vi "HFRR ADV v01.vi"() -> ()   [LabVIEW 2025] (continued)
            n1565 = Concatenate Strings("(" ("string"), w1652, " ) % RH," ("string")) -> (w1651:string)
            n1566 = Concatenate Strings("(" ("string"), w1648, ")  Deg C ," ("string")) -> (w1647:string)
            n1567 = Concatenate Strings("(" ("string"), w1645, ")  Microns," ("string")) -> (w1644:string)
            n1568 = Concatenate Strings("(" ("string"), w1641, ")  kPa," ("string")) -> (w1631:string)
            n1569 = Concatenate Strings(w1685, ".dwm" ("Substring")) -> (w1683:string)
            n1570 = String To Path(string=w1683) -> (path=w1682:path)
            n1571 = Concatenate Strings(w1665, w1630, " Humidity before test= " ("Substring"), w1660, w1630, " Temperature before test = " ("Substring"), w1655, w1630, " Humidity after test= " ("Substring"), w1651, w1630, "Temperature after test = " ("Substring"), w1647, w1630, "MSD = " ("Substring"), w1644, w1630, "  AVP = " ("Substring"), w1631, w1630, "  HCF                     =( " ("Substring"), w1637, w1630, " WS1.4                  = " ("Substring"), w1633, w1630) -> (w1629:string)
            "data" <- w1629
            n1572 = call <vilib>:"Write Characters To File.vi"("append to file? (new file:F)"=FALSE, "character string"=w1629, "file path (dialog if empty)"=w1682) -> ()  [unwired: 2 in, 1 out]
            n1573 = Match Pattern(string=w1629, regular expression="!") -> (after substring=→"export":string)  [unwired: 1 in, 3 out]
          }
        }
        n1574 = Add(x=231.864, y=w1601) -> (x+y=w1598:dbl)
        n1575 = Add(x=231.864, y=w1614) -> (x+y=w1611:dbl)
        n1576 = Divide(x=1705.984, y=w1598) -> (x/y=w1599:dbl)
        n1577 = Divide(x=1705.984, y=w1611) -> (x/y=w1612:dbl)
        n1578 = local read "Humidity before test"() -> (w1603:dbl)
        n1579 = local read "Humidity after test"() -> (w1616:dbl)
        n1580 = Subtract(x=8.017352 ("y"), y=w1599) -> (x-y=w1625:dbl)
        n1581 = Subtract(x=8.017352 ("y"), y=w1612) -> (x-y=w1619:dbl)
        n1582 = expression code="10**y"(w1625) -> (w1605:dbl)
        n1583 = expression code="10**y"(w1619) -> (w1618:dbl)
        n1584 = Multiply(x=w1603, y=w1605) -> (x*y=w1604:dbl)
        n1585 = Multiply(x=w1616, y=w1618) -> (x*y=w1617:dbl)
        n1586 = Divide(x=w1604, y=750.0) -> (x/y=w1620:dbl)
        n1587 = Divide(x=w1617, y=750.0) -> (x/y=w1621:dbl)
        n1588 = Add(x=w1620, y=w1621) -> (x+y=w1622:dbl)
        n1589 = Divide(x=w1622, y=2.0) -> (x/y=w1624:dbl)
        n1590 = local write "AVP"(w1624) -> ()
        n1591 = Subtract(x=1.4, y=w1624) -> (x-y=w1607:dbl)
        n1592 = local read "HCF"() -> (w1608:dbl)
      }
      frame Enabled {
      }
    }
    n1593 = case shown="True" "EDIT 3" {
      frame False {
      }
      frame True {
        n1594 = local write "EDIT 3"(FALSE ("EDIT 3")) -> ()
        n1595 = local write "Main Tab"(T2."About" ("Main Tab")) -> ()
      }
    }
    n1596 = case shown="True" w1579 {
      frame False {
      }
      frame True {
        n1597 = local write "Re-Initialise"(FALSE ("Re-Initialise")) -> ()
      }
    }
    n1598 = case shown="False" w1593 {
      frame False {
        n1599 = local read "stopT"() -> (w2573:bool)
        n1600 = case shown="True" w2573 {
          frame False {
          }
          frame True {
            n1601 = local write "stopT"(FALSE) -> ()
          }
        }
      }
      frame True {
        "stopT" <- TRUE
      }
    }
    n1602 = case shown="False" w1591 {
      frame False {
      }
      frame True {
      }
    }
    n1603 = case shown="True" w1581 {
      frame False {
        n1604 = property on="Password 2" class="Str"("Visible"=FALSE) -> ()  [unwired: 2 in, 2 out]
        n1605 = local write "Password 2"("" ("Password")) -> ()
      }
      frame True {
        n1606 = property on="Password 2" class="Str"("Visible"=TRUE) -> ()  [unwired: 2 in, 2 out]
        n1607 = Equal?(x="Password 2", y="HFRR1234") -> (x = y?=w1714:bool)
        n1608 = case shown="True" w1714 {
          tunnel: "Password 2" -> [w1717 _]
          frame False {
            n1609 = String Length(string=w1717) -> (length=w1718:i32)
            n1610 = Greater Than 0?(x=w1718) -> (x > 0?=w1716:bool)
            n1611 = case shown="False" w1716 {
              frame False {
                n1612 = property on="Password 2" class="Str"("Caption.Text"="Password (Advance Setting)") -> ()  [unwired: 2 in, 2 out]
              }
              frame True {
                n1613 = property on="Password 2" class="Str"("Caption.Text"="Incorrect Password!") -> ()  [unwired: 2 in, 2 out]
              }
            }
          }
          frame True {
            n1614 = local write "EDIT 2"(FALSE ("EDIT 2")) -> ()
            n1615 = local write "Password 2"("" ("Password")) -> ()
            n1616 = local write "Main Tab"(T2."Advance" ("Main Tab")) -> ()
            n1617 = local write "Main Dashboard Buttons"(T1."Advance" ("Main Dashboard Buttons")) -> ()
          }
        }
      }
    }
    n1618 = case shown="True" "Prog Uno" {
      frame False {
      }
      frame True {
        n1619 = stacked-sequence {
          frame #0 {
            n1620 = Delete(path (use dialog)=path "C:/LAB-IQ-NXT/UNOCOMPILE.bat" ("working directory")) -> ()  [unwired: 4 in, 3 out]
          }
          frame #1 {
            n1621 = local read "Com Port 1"() -> (w2179:refnum<visa-resource-name>)
            n1622 = Concatenate Strings("cmd.exe /c \"mode " ("command line"), w2179, ":1200,n,8,1\"\n" ("command line")) -> (w2184:string)
            n1623 = Concatenate Strings(w2184, "CD\\\nCD WinDucom\navrdude -C avrdude.conf -v -patmega328p -carduino -P" ("command line"), w2179, " -b115200 -D -Uflash:w:UNO_V20.hex:i\n" ("command line"), "\r") -> (w2186:string)
            "STR" <- w2186
            n1624 = call <vilib>:"Write Characters To File.vi"("append to file? (new file:F)"=FALSE, "character string"=w2186, "file path (dialog if empty)"=path "C:/LAB-IQ/UNOCOMPILE.bat" ("working directory")) -> ()  [unwired: 2 in, 1 out]
          }
          frame #2 {
            n1625 = disable-structure shown="Disabled" {
              frame Disabled {
                w2190 = "cmd.exe  /c \"C:\\LAB-IQ-NXT\\UNOCOMPILE.bat\"" ("string")
                n1626 = local write "Prog Uno"(FALSE ("run minimized? (F)")) -> ()
                n1627 = call <vilib>:"System Exec.vi"("expected output size  (4096)"=u32 65535, "run minimized? (F)"=FALSE, "wait until completion? (T)"=TRUE ("run minimized? (F)"), "working directory"=path "C:/LAB-IQ-NXT", "standard input"=w2190, "command line"=w2190) -> ("error out"=w2189:errorcluster, "standard output"=→"String 42":string)  [unwired: 2 in, 2 out]
                "error out 3" <- w2189
                n1628 = flat-sequence {
                  tunnel: w2189 -> [_]
                  frame #0 {
                  }
                }
              }
              frame Enabled {
              }
            }
          }
        }
      }
    }
    n1629 = case shown="\"CEC F-096-A-06\"" "TEST STANDARD" {
      tunnel: [2.0 ("Set Temp") 0.0 ("Set Temp") 2.0 ("Set Temp") 0.0 ("Set Temp")] -> w1582
      frame "ASTM D6079", Default {
        w2136 = 50.0 ("Hz")
        w2137 = 53.0 ("Set Rh")
        w2139 = 1.0 ("Set Strk")
        w2138 = 60.0 ("Set Temp")
        # "astm hide"
        n1630 = local write "NORMAL LOAD"(200.0 ("NORMAL LOAD")) -> ()
        n1631 = local write "Set Strk"(w2139) -> ()
        n1632 = local write "Set Hz"(w2136) -> ()
        n1633 = local write "Set Temp"(w2138) -> ()
        n1634 = local write "Set Rh"(w2137) -> ()
        n1635 = local write "test time"(75.0 ("test time")) -> ()
        n1636 = local write "Set Stroke:"(w2139) -> ()
        n1637 = local write "Set Humidity:"(w2137) -> ()
        n1638 = local write "Set Frequency:"(w2136) -> ()
        n1639 = local write "Set Temperature:"(w2138) -> ()
        "Test Standard" <- "ASTM D6079" ("Test Standard 2")
      }
      frame "ISO 12156" {
        n1640 = local write "Set Strk"(1.0 ("Set Strk")) -> ()
        n1641 = local write "NORMAL LOAD"(200.0 ("NORMAL LOAD")) -> ()
        n1642 = local write "Set Temp"(60.0 ("Set Temp")) -> ()
        n1643 = local write "test time"(75.0 ("test time")) -> ()
        n1644 = local write "Set Hz"(50.0 ("Hz")) -> ()
        n1645 = local write "Set Rh"(53.0 ("Set Rh")) -> ()
      }
      frame "CEC F-096-A-06" {
        n1646 = local write "Set Strk"(1.0 ("Set Strk")) -> ()
        n1647 = local write "NORMAL LOAD"(200.0 ("NORMAL LOAD")) -> ()
        n1648 = local write "Set Temp"(60.0 ("Set Temp")) -> ()
        n1649 = local write "test time"(75.0 ("test time")) -> ()
        n1650 = local write "Set Hz"(50.0 ("Hz")) -> ()
        n1651 = local write "Set Rh"(53.0 ("Set Rh")) -> ()
      }
      frame "Custom" {
      }
    }
    n1652 = case shown="True" "Prog Due" {
      frame False {
      }
      frame True {
        n1653 = stacked-sequence {
          frame #0 {
            n1654 = Delete(path (use dialog)=path "C:/LAB-IQ/DUECOMPILE.bat" ("working directory")) -> ()  [unwired: 4 in, 3 out]
          }
          frame #1 {
            n1655 = disable-structure shown="Disabled" {
              frame Disabled {
                n1656 = local read "visa due"() -> (w2161:string)
                n1657 = Concatenate Strings("cmd.exe /c \"mode " ("command line"), w2161, ":1200,n,8,1\"\n" ("command line")) -> (w2166:string)
                n1658 = Concatenate Strings(w2166, "CD\\\nCD WinDucom\nTIMEOUT 1\n bossac.exe -i -d --port=" ("command line"), w2161, " -U false -e -w -v -b DUE.bin -R\n" ("command line"), "\r") -> (w2168:string)
                "concatenated string 2" <- w2168
                n1659 = call <vilib>:"Write Characters To File.vi"("append to file? (new file:F)"=FALSE, "character string"=w2168, "file path (dialog if empty)"=path "C:/LAB-IQ-NXT/DUECOMPILE.bat" ("working directory")) -> ()  [unwired: 2 in, 1 out]
              }
              frame Enabled {
              }
            }
          }
          frame #2 {
            # "C:\\LAB-IQ-NXT\\DUECOMPILE.bat"
            n1660 = disable-structure shown="Disabled" {
              frame Disabled {
                w2173 = "cmd.exe  /c \"C:\\LAB-IQ-NXT\\DUECOMPILE.bat\"" ("string")
                n1661 = call <vilib>:"System Exec.vi"("expected output size  (4096)"=u32 65535, "run minimized? (F)"=FALSE, "wait until completion? (T)"=TRUE ("run minimized? (F)"), "working directory"=path "C:/LAB-IQ-NXT", "standard input"=w2173, "command line"=w2173) -> ("error out"=w2172:errorcluster, "standard output"=→"String 44":string)  [unwired: 2 in, 2 out]
                "error out 4" <- w2172
                n1662 = flat-sequence {
                  tunnel: w2172 -> [_]
                  frame #0 {
                  }
                }
              }
              frame Enabled {
              }
            }
            n1663 = local write "Prog Due"(FALSE ("Prog Due")) -> ()
          }
        }
      }
    }
    n1664 = Or(x=w1578, y=w1576) -> (x .or. y?=w1577:bool)
    n1665 = case shown="\"About\"" w1575 {
      tunnel: [T22."Acquire" ("Main Tab") T22."Compare Files" ("Main Tab") T22."About" ("Main Tab")] -> w1589
      frame "Acquire", Default {
      }
      frame "Compare Files" {
      }
      frame "About" {
      }
    }
    n1666 = Or(x=w1583, y="OPEN") -> (x .or. y?=w1584:bool)
    n1667 = case shown="True" w1584 {
      tunnel: w1583 -> [_ w1725]
      frame False {
      }
      frame True {
        n1668 = stacked-sequence {
          tunnel: w1725 -> [_ w1792 _ _]
          frame #0 {
            w1741 = "  " ("String 6")
            n1669 = local write "OPEN"(FALSE ("open")) -> ()
            n1670 = local read "string1 2"() -> (w1729:string)
            n1671 = local read "string1 3"() -> (w1728:string)
            n1672 = local read "string1 4"() -> (w1727:string)
            n1673 = property on="OPEN" class="Bool (strict)"("Visible"=FALSE) -> ()  [unwired: 2 in, 2 out]
            n1674 = local write "String 6"(w1741) -> ()
            n1675 = local write "String 7"(w1741) -> ()
            n1676 = local write "String 8"(w1741) -> ()
            n1677 = local write "String 12"(w1741) -> ()
            n1678 = local read "OK Button 16"() -> (w1726:bool)
            n1679 = String To Path(string=w1729) -> (path=w1737:path)
            n1680 = String To Path(string=w1728) -> (path=w1736:path)
            n1681 = String To Path(string=w1727) -> (path=w1735:path)
            n1682 = case shown="True" w1726 {
              tunnel: [w1742 w1743] -> w1730
              frame False {
                n1683 = local read "string1"() -> (w1742:string)
              }
              frame True {
                n1684 = local read "String Indicator 4"() -> (w1743:string)
              }
            }
            n1685 = Open/Create/Replace File "Open File"(file path (use dialog)=w1737) -> (refnum out=w1733:refnum<file>)  [unwired: 5 in, 2 out]
            n1686 = Open/Create/Replace File "Open File"(file path (use dialog)=w1736) -> (refnum out=w1732:refnum<file>)  [unwired: 5 in, 2 out]
            n1687 = Open/Create/Replace File "Open File"(file path (use dialog)=w1735) -> (refnum out=w1731:refnum<file>)  [unwired: 5 in, 2 out]
            n1688 = while {
              tunnel: w1733 -> [w1755]
              i -> [w1751]
              stop <- w1750 continue-if-true
              (unwired) TRUE ("line mode (F)")
              n1689 = Read from Text File "Read File"(file (use dialog)=w1755) -> (text=w1752:string)  [unwired: 3 in, 3 out]
              n1690 = local write "Numeric 11"(w1751) -> ()
              n1691 = String Length(string=w1752) -> (length=w1754:i32)
              n1692 = Greater?(x=w1754, y=1) -> (0:w1750:bool)
            }
            n1693 = while {
              tunnel: w1732 -> [w1761]
              i -> [w1757]
              stop <- w1756 continue-if-true
              (unwired) TRUE ("line mode (F)")
              n1694 = Read from Text File "Read File"(file (use dialog)=w1761) -> (text=w1758:string)  [unwired: 3 in, 3 out]
              n1695 = local write "Numeric 12"(w1757) -> ()
              n1696 = String Length(string=w1758) -> (length=w1760:i32)
              n1697 = Greater?(x=w1760, y=1) -> (0:w1756:bool)
            }
            n1698 = while {
              tunnel: w1731 -> [w1767]
              i -> [w1763]
              stop <- w1762 continue-if-true
              (unwired) TRUE ("line mode (F)")
              n1699 = Read from Text File "Read File"(file (use dialog)=w1767) -> (text=w1764:string)  [unwired: 3 in, 3 out]
              n1700 = local write "Numeric 13"(w1763) -> ()
              n1701 = String Length(string=w1764) -> (length=w1766:i32)
              n1702 = Greater?(x=w1766, y=1) -> (0:w1762:bool)
            }
            n1703 = String To Path(string=w1730) -> (path=w1738:path)
            n1704 = Open/Create/Replace File "Open File"(file path (use dialog)=w1738) -> (refnum out=w1734:refnum<file>)  [unwired: 5 in, 2 out]
            n1705 = while {
              tunnel: w1734 -> [w1749]
              i -> [w1745]
              stop <- w1744 continue-if-true
              (unwired) TRUE ("line mode (F)")
              n1706 = Read from Text File "Read File"(file (use dialog)=w1749) -> (text=w1746:string)  [unwired: 3 in, 3 out]
              n1707 = local write "Numeric 8"(w1745) -> ()
              n1708 = String Length(string=w1746) -> (length=w1748:i32)
              n1709 = Greater?(x=w1748, y=1) -> (0:w1744:bool)
            }
          }
          frame #1 {
            w1919 = FALSE ("ACTUAL   MERGE")
            # "Sample Temp"
            # "ECR"
            # "COF"
            # "Time\nCOF\nFF\nTemp"
            n1710 = case shown="True" w1792 {
              tunnel: [w1939 w1940] -> w1793
              frame False {
                n1711 = local read "string1"() -> (w1939:string)
              }
              frame True {
                n1712 = local read "String Indicator 4"() -> (w1940:string)
              }
            }
            n1713 = local read "string1 3"() -> (w1837:string)
            n1714 = String To Path(string=w1793) -> (path=w1924:path)
            n1715 = String To Path(string=w1837) -> (path=w1935:path)
            n1716 = local read "Numeric 12"() -> (w1921:i32)
            n1717 = local read "Numeric 8"() -> (w1923:i32)
            n1718 = local read "string1 2"() -> (w1838:string)
            n1719 = local read "string1 4"() -> (w1836:string)
            n1720 = Open/Create/Replace File "Open File"(file path (use dialog)=w1924) -> (refnum out=w1938:refnum<file>, error out=w1937:errorcluster)  [unwired: 5 in, 1 out]
            n1721 = Open/Create/Replace File "Open File"(file path (use dialog)=w1935) -> (refnum out=w1931:refnum<file>, error out=w1932:errorcluster)  [unwired: 5 in, 1 out]
            n1722 = for {
              N: w1923 -> [_]
              tunnel: w1938 -> [w2086]
              tunnel: w1937 -> [w2085]
              tunnel: [w2075] -> w1850 mode=indexing
              tunnel: [w2073] -> w1907 mode=indexing
              tunnel: [w2074] -> w1902 mode=indexing
              tunnel: w1919 -> [_]
              tunnel: [w2067] -> w1904 mode=indexing
              tunnel: [w2063] -> w1873 mode=indexing
              tunnel: [w2059] -> w1848 mode=indexing
              tunnel: [w2055] -> w1829 mode=indexing
              tunnel: [w2050] -> w1789 mode=indexing
              (unwired) TRUE ("line mode (F)")
              # "freq"
              # "Stroke"
              # "Time"
              # "CoF"
              # "Humidity"
              # "Temp"
              # "Air Temp"
              # "ECR"
              n1723 = Read from Text File "Read File"(file (use dialog)=w2086, error in=w2085) -> (text=w2051:string)  [unwired: 2 in, 3 out]
              n1724 = local write "String 6"(w2051) -> ()
              n1725 = String Subset(string=w2051, offset (0)=0, length (rest)=14 ("length (rest)")) -> (substring=w2079:string)
              n1726 = String Subset(string=w2051, offset (0)=35, length (rest)=9 ("length (rest)")) -> (substring=w2076:string)
              n1727 = String Subset(string=w2051, offset (0)=15, length (rest)=9 ("length (rest)")) -> (substring=w2082:string)
              n1728 = Fract/Exp String To Number(string=w2079) -> (number=w2075:dbl)  [unwired: 3 in, 1 out]
              n1729 = Fract/Exp String To Number(string=w2076) -> (number=w2074:dbl)  [unwired: 3 in, 1 out]
              n1730 = Fract/Exp String To Number(string=w2082) -> (number=w2073:dbl)  [unwired: 3 in, 1 out]
              n1731 = String Subset(string=w2051, offset (0)=85, length (rest)=9 ("length (rest)")) -> (substring=w2052:string)
              n1732 = String Subset(string=w2051, offset (0)=25, length (rest)=9 ("length (rest)")) -> (substring=w2058:string)
              n1733 = String Subset(string=w2051, offset (0)=55, length (rest)=9 ("length (rest)")) -> (substring=w2060:string)
              n1734 = String Subset(string=w2051, offset (0)=45, length (rest)=9 ("length (rest)")) -> (substring=w2066:string)
              n1735 = String Subset(string=w2051, offset (0)=65, length (rest)=9 ("length (rest)")) -> (substring=w2072:string)
              n1736 = Fract/Exp String To Number(string=w2058) -> (number=w2055:dbl)  [unwired: 3 in, 1 out]
              n1737 = Fract/Exp String To Number(string=w2052) -> (number=w2050:dbl)  [unwired: 3 in, 1 out]
              n1738 = Fract/Exp String To Number(string=w2060) -> (number=w2059:dbl)  [unwired: 3 in, 1 out]
              n1739 = Fract/Exp String To Number(string=w2066) -> (number=w2063:dbl)  [unwired: 3 in, 1 out]
              n1740 = Fract/Exp String To Number(string=w2072) -> (number=w2069:dbl)  [unwired: 3 in, 1 out]
              n1741 = Add(x=w2069, y=0.0) -> (x+y=w2067:dbl)
            }
            n1742 = for {
              N: w1921 -> [_]
              tunnel: w1932 -> [w2012]
              tunnel: w1931 -> [w2011]
              tunnel: [w2001] -> w1890 mode=indexing
              tunnel: [w1999] -> w1888 mode=indexing
              tunnel: [w2000] -> w1884 mode=indexing
              tunnel: w1919 -> [_]
              tunnel: [w1993] -> w1886 mode=indexing
              tunnel: [w1989] -> w1868 mode=indexing
              tunnel: [w1985] -> w1844 mode=indexing
              tunnel: [w1982] -> w1825 mode=indexing
              tunnel: [w1978] -> w1784 mode=indexing
              (unwired) 9 ("length (rest)")
              (unwired) 9 ("length (rest)")
              (unwired) TRUE ("line mode (F)")
              n1743 = Read from Text File "Read File"(file (use dialog)=w2011, error in=w2012) -> (text=w1979:string)  [unwired: 2 in, 3 out]
              n1744 = local write "String 8"(w1979) -> ()
              n1745 = String Subset(string=w1979, offset (0)=85) -> (substring=w1981:string)  [unwired: 1 in]
              n1746 = String Subset(string=w1979, offset (0)=35, length (rest)=9 ("length (rest)")) -> (substring=w2002:string)
              n1747 = String Subset(string=w1979, offset (0)=55, length (rest)=9 ("length (rest)")) -> (substring=w1987:string)
              n1748 = String Subset(string=w1979, offset (0)=25) -> (substring=w1983:string)  [unwired: 1 in]
              n1749 = String Subset(string=w1979, offset (0)=15, length (rest)=9 ("length (rest)")) -> (substring=w2008:string)
              n1750 = String Subset(string=w1979, offset (0)=0, length (rest)=14 ("length (rest)")) -> (substring=w2005:string)
              n1751 = String Subset(string=w1979, offset (0)=45, length (rest)=9 ("length (rest)")) -> (substring=w1992:string)
              n1752 = String Subset(string=w1979, offset (0)=65, length (rest)=9 ("length (rest)")) -> (substring=w1998:string)
              n1753 = Fract/Exp String To Number(string=w1981) -> (number=w1978:dbl)  [unwired: 3 in, 1 out]
              n1754 = Fract/Exp String To Number(string=w2002) -> (number=w2000:dbl)  [unwired: 3 in, 1 out]
              n1755 = Fract/Exp String To Number(string=w1987) -> (number=w1985:dbl)  [unwired: 3 in, 1 out]
              n1756 = Fract/Exp String To Number(string=w1983) -> (number=w1982:dbl)  [unwired: 3 in, 1 out]
              n1757 = Fract/Exp String To Number(string=w2008) -> (number=w1999:dbl)  [unwired: 3 in, 1 out]
              n1758 = Fract/Exp String To Number(string=w2005) -> (number=w2001:dbl)  [unwired: 3 in, 1 out]
              n1759 = Fract/Exp String To Number(string=w1992) -> (number=w1989:dbl)  [unwired: 3 in, 1 out]
              n1760 = Fract/Exp String To Number(string=w1998) -> (number=w1995:dbl)  [unwired: 3 in, 1 out]
              n1761 = Add(x=w1995, y=0.0) -> (x+y=w1993:dbl)
            }
            n1762 = String To Path(string=w1838) -> (path=w1936:path)
            n1763 = String To Path(string=w1836) -> (path=w1930:path)
            n1764 = local read "Numeric 11"() -> (w1920:i32)
            n1765 = local read "Numeric 13"() -> (w1922:i32)
            n1766 = Open/Create/Replace File "Open File"(file path (use dialog)=w1936) -> (refnum out=w1934:refnum<file>, error out=w1933:errorcluster)  [unwired: 5 in, 1 out]
            n1767 = Open/Create/Replace File "Open File"(file path (use dialog)=w1930) -> (refnum out=w1929:refnum<file>, error out=w1928:errorcluster)  [unwired: 5 in, 1 out]
            n1768 = for {
              N: w1920 -> [_]
              tunnel: w1934 -> [w2049]
              tunnel: w1933 -> [w2048]
              tunnel: [w2038] -> w1900 mode=indexing
              tunnel: [w2036] -> w1898 mode=indexing
              tunnel: [w2037] -> w1893 mode=indexing
              tunnel: w1919 -> [_]
              tunnel: [w2030] -> w1895 mode=indexing
              tunnel: [w2026] -> w1871 mode=indexing
              tunnel: [w2022] -> w1846 mode=indexing
              tunnel: [w2018] -> w1827 mode=indexing
              tunnel: [w2013] -> w1785 mode=indexing
              (unwired) TRUE ("line mode (F)")
              n1769 = Read from Text File "Read File"(file (use dialog)=w2049, error in=w2048) -> (text=w2014:string)  [unwired: 2 in, 3 out]
              n1770 = local write "String 7"(w2014) -> ()
              n1771 = String Subset(string=w2014, offset (0)=85, length (rest)=9 ("length (rest)")) -> (substring=w2017:string)
              n1772 = String Subset(string=w2014, offset (0)=35, length (rest)=9 ("length (rest)")) -> (substring=w2039:string)
              n1773 = String Subset(string=w2014, offset (0)=55, length (rest)=9 ("length (rest)")) -> (substring=w2025:string)
              n1774 = String Subset(string=w2014, offset (0)=25, length (rest)=9 ("length (rest)")) -> (substring=w2019:string)
              n1775 = String Subset(string=w2014, offset (0)=45, length (rest)=9 ("length (rest)")) -> (substring=w2027:string)
              n1776 = String Subset(string=w2014, offset (0)=0, length (rest)=14 ("length (rest)")) -> (substring=w2042:string)
              n1777 = String Subset(string=w2014, offset (0)=15, length (rest)=9 ("length (rest)")) -> (substring=w2045:string)
              n1778 = String Subset(string=w2014, offset (0)=65, length (rest)=9 ("length (rest)")) -> (substring=w2031:string)
              n1779 = Fract/Exp String To Number(string=w2017) -> (number=w2013:dbl)  [unwired: 3 in, 1 out]
              n1780 = Fract/Exp String To Number(string=w2039) -> (number=w2037:dbl)  [unwired: 3 in, 1 out]
              n1781 = Fract/Exp String To Number(string=w2025) -> (number=w2022:dbl)  [unwired: 3 in, 1 out]
              n1782 = Fract/Exp String To Number(string=w2019) -> (number=w2018:dbl)  [unwired: 3 in, 1 out]
              n1783 = Fract/Exp String To Number(string=w2027) -> (number=w2026:dbl)  [unwired: 3 in, 1 out]
              n1784 = Fract/Exp String To Number(string=w2042) -> (number=w2038:dbl)  [unwired: 3 in, 1 out]
              n1785 = Fract/Exp String To Number(string=w2045) -> (number=w2036:dbl)  [unwired: 3 in, 1 out]
              n1786 = Fract/Exp String To Number(string=w2031) -> (number=w2034:dbl)  [unwired: 3 in, 1 out]
              n1787 = Add(x=w2034, y=0.0) -> (x+y=w2030:dbl)
            }
            n1788 = for {
              N: w1922 -> [_]
              tunnel: w1929 -> [w1977]
              tunnel: w1928 -> [w1976]
              tunnel: [w1966] -> w1882 mode=indexing
              tunnel: [w1965] -> w1875 mode=indexing
              tunnel: w1919 -> [_]
              tunnel: [w1954] -> w1880 mode=indexing
              tunnel: [w1959] -> w1877 mode=indexing
              tunnel: [w1955] -> w1867 mode=indexing
              tunnel: [w1950] -> w1842 mode=indexing
              tunnel: [w1946] -> w1823 mode=indexing
              tunnel: [w1941] -> w1783 mode=indexing
              (unwired) 1.0 ("x")
              (unwired) TRUE ("line mode (F)")
              n1789 = Read from Text File "Read File"(file (use dialog)=w1977, error in=w1976) -> (text=w1942:string)  [unwired: 2 in, 3 out]
              n1790 = local write "String 12"(w1942) -> ()
              n1791 = String Subset(string=w1942, offset (0)=85, length (rest)=9 ("length (rest)")) -> (substring=w1944:string)
              n1792 = String Subset(string=w1942, offset (0)=35, length (rest)=9 ("length (rest)")) -> (substring=w1967:string)
              n1793 = String Subset(string=w1942, offset (0)=55, length (rest)=9 ("length (rest)")) -> (substring=w1952:string)
              n1794 = String Subset(string=w1942, offset (0)=25, length (rest)=9 ("length (rest)")) -> (substring=w1948:string)
              n1795 = String Subset(string=w1942, offset (0)=45, length (rest)=9 ("length (rest)")) -> (substring=w1957:string)
              n1796 = String Subset(string=w1942, offset (0)=15, length (rest)=9 ("length (rest)")) -> (substring=w1973:string)
              n1797 = String Subset(string=w1942, offset (0)=0, length (rest)=14 ("length (rest)")) -> (substring=w1970:string)
              n1798 = String Subset(string=w1942, offset (0)=65, length (rest)=9 ("length (rest)")) -> (substring=w1960:string)
              n1799 = Fract/Exp String To Number(string=w1944) -> (number=w1941:dbl)  [unwired: 3 in, 1 out]
              n1800 = Fract/Exp String To Number(string=w1967) -> (number=w1965:dbl)  [unwired: 3 in, 1 out]
              n1801 = Fract/Exp String To Number(string=w1952) -> (number=w1950:dbl)  [unwired: 3 in, 1 out]
              n1802 = Fract/Exp String To Number(string=w1948) -> (number=w1946:dbl)  [unwired: 3 in, 1 out]
              n1803 = Fract/Exp String To Number(string=w1957) -> (number=w1955:dbl)  [unwired: 3 in, 1 out]
              n1804 = Fract/Exp String To Number(string=w1973) -> (number=w1954:dbl)  [unwired: 3 in, 1 out]
              n1805 = Fract/Exp String To Number(string=w1970) -> (number=w1966:dbl)  [unwired: 3 in, 1 out]
              n1806 = Fract/Exp String To Number(string=w1960) -> (number=w1963:dbl)  [unwired: 3 in, 1 out]
              n1807 = Add(x=w1963, y=0.0) -> (x+y=w1959:dbl)
            }
            n1808 = Delete From Array(array=w1825, index=0) -> (array with subset deleted=w1798:dbl[])  [unwired: 1 in, 1 out]
            n1809 = Delete From Array(array=w1888, index=0) -> (array with subset deleted=w1861:dbl[])  [unwired: 1 in, 1 out]
            n1810 = Delete From Array(array=w1868, index=0) -> (array with subset deleted=w1856:dbl[])  [unwired: 1 in, 1 out]
            n1811 = Delete From Array(array=w1886, index=0) -> (array with subset deleted=w1887:dbl[])  [unwired: 1 in, 1 out]
            n1812 = call-poly <vilib>:"Mean.vi"("X"=w1798) -> ("mean"=→"КОФ2 4":dbl)  [unwired: 1 out]
            n1813 = call-poly <vilib>:"Mean.vi"("X"=w1861) -> ("mean"=→"КОФ3":dbl)  [unwired: 1 out]
            n1814 = call-poly <vilib>:"Mean.vi"("X"=w1856) -> ("mean"=→"CP3":dbl)  [unwired: 1 out]
            n1815 = Delete From Array(array=w1850, index=0) -> (array with subset deleted=w1777:dbl[])  [unwired: 1 in, 1 out]
            n1816 = Delete From Array(array=w1789, index=0) -> (array with subset deleted=w1776:dbl[])  [unwired: 1 in, 1 out]
            n1817 = Delete From Array(array=w1829, index=0) -> (array with subset deleted=w1800:dbl[])  [unwired: 1 in, 1 out]
            n1818 = Delete From Array(array=w1907, index=0) -> (array with subset deleted=w1862:dbl[])  [unwired: 1 in, 1 out]
            n1819 = Delete From Array(array=w1873, index=0) -> (array with subset deleted=w1858:dbl[])  [unwired: 1 in, 1 out]
            "array w/ subset deleted" <- w1858
            n1820 = Delete From Array(array=w1904, index=0) -> (array with subset deleted=w1905:dbl[])  [unwired: 1 in, 1 out]
            n1821 = call-poly <vilib>:"Mean.vi"("X"=w1800) -> ("mean"=→"КОФ2 2":dbl)  [unwired: 1 out]
            n1822 = call-poly <vilib>:"Mean.vi"("X"=w1862) -> ("mean"=→"КОФ1":dbl)  [unwired: 1 out]
            n1823 = Bundle "Bundle"(w1777, w1776) -> (w1782:cluster{dbl[], dbl[]})  [unwired: 1 in]
            n1824 = Bundle "Bundle"(w1777, w1905) -> (w1769:cluster{dbl[], dbl[]})  [unwired: 1 in]
            n1825 = Delete From Array(array=w1784, index=0) -> (array with subset deleted=w1772:dbl[])  [unwired: 1 in, 1 out]
            n1826 = Delete From Array(array=w1785, index=0) -> (array with subset deleted=w1774:dbl[])  [unwired: 1 in, 1 out]
            n1827 = Delete From Array(array=w1895, index=0) -> (array with subset deleted=w1896:dbl[])  [unwired: 1 in, 1 out]
            n1828 = Delete From Array(array=w1783, index=0) -> (array with subset deleted=w1770:dbl[])  [unwired: 1 in, 1 out]
            n1829 = Delete From Array(array=w1877, index=0) -> (array with subset deleted=w1878:dbl[])  [unwired: 1 in, 1 out]
            n1830 = Delete From Array(array=w1902, index=0) -> (array with subset deleted=w1808:dbl[])  [unwired: 1 in, 1 out]
            n1831 = Delete From Array(array=w1848, index=0) -> (array with subset deleted=w1804:dbl[])  [unwired: 1 in, 1 out]
            n1832 = Delete From Array(array=w1884, index=0) -> (array with subset deleted=w1806:dbl[])  [unwired: 1 in, 1 out]
            n1833 = Delete From Array(array=w1844, index=0) -> (array with subset deleted=w1802:dbl[])  [unwired: 1 in, 1 out]
            n1834 = Delete From Array(array=w1893, index=0) -> (array with subset deleted=w1807:dbl[])  [unwired: 1 in, 1 out]
            n1835 = Delete From Array(array=w1846, index=0) -> (array with subset deleted=w1803:dbl[])  [unwired: 1 in, 1 out]
            n1836 = Delete From Array(array=w1827, index=0) -> (array with subset deleted=w1799:dbl[])  [unwired: 1 in, 1 out]
            n1837 = Delete From Array(array=w1871, index=0) -> (array with subset deleted=w1857:dbl[])  [unwired: 1 in, 1 out]
            n1838 = Delete From Array(array=w1898, index=0) -> (array with subset deleted=w1859:dbl[])  [unwired: 1 in, 1 out]
            n1839 = Delete From Array(array=w1875, index=0) -> (array with subset deleted=w1805:dbl[])  [unwired: 1 in, 1 out]
            n1840 = Delete From Array(array=w1842, index=0) -> (array with subset deleted=w1801:dbl[])  [unwired: 1 in, 1 out]
            n1841 = Delete From Array(array=w1823, index=0) -> (array with subset deleted=w1797:dbl[])  [unwired: 1 in, 1 out]
            n1842 = Delete From Array(array=w1867, index=0) -> (array with subset deleted=w1855:dbl[])  [unwired: 1 in, 1 out]
            n1843 = Delete From Array(array=w1880, index=0) -> (array with subset deleted=w1860:dbl[])  [unwired: 1 in, 1 out]
            n1844 = Delete From Array(array=w1890, index=0) -> (array with subset deleted=w1773:dbl[])  [unwired: 1 in, 1 out]
            n1845 = Delete From Array(array=w1900, index=0) -> (array with subset deleted=w1775:dbl[])  [unwired: 1 in, 1 out]
            n1846 = Delete From Array(array=w1882, index=0) -> (array with subset deleted=w1771:dbl[])  [unwired: 1 in, 1 out]
            n1847 = Bundle "Bundle"(w1777, w1808) -> (w1795:cluster{dbl[], dbl[]})  [unwired: 1 in]
            n1848 = Bundle "Bundle"(w1777, w1862) -> (w1796:cluster{dbl[], dbl[]})  [unwired: 1 in]
            n1849 = Bundle "Bundle"(w1808, w1804) -> (w1810:cluster{dbl[], dbl[]})  [unwired: 1 in]
            n1850 = Bundle "Bundle"(w1773, w1772) -> (w1780:cluster{dbl[], dbl[]})  [unwired: 1 in]
            n1851 = Bundle "Bundle"(w1806, w1802) -> (w1812:cluster{dbl[], dbl[]})  [unwired: 1 in]
            n1852 = Bundle "Bundle"(w1773, w1806) -> (w1916:cluster{dbl[], dbl[]})  [unwired: 1 in]
            n1853 = Bundle "Bundle"(w1773, w1802) -> (w1840:cluster{dbl[], dbl[]})  [unwired: 1 in]
            n1854 = Bundle "Bundle"(w1773, w1861) -> (w1926:cluster{dbl[], dbl[]})  [unwired: 1 in]
            n1855 = Bundle "Bundle"(w1773, w1856) -> (w1864:cluster{dbl[], dbl[]})  [unwired: 1 in]
            n1856 = Bundle "Bundle"(w1773, w1887) -> (w1911:cluster{dbl[], dbl[]})  [unwired: 1 in]
            n1857 = Bundle "Bundle"(w1807, w1803) -> (w1811:cluster{dbl[], dbl[]})  [unwired: 1 in]
            n1858 = Bundle "Bundle"(w1775, w1774) -> (w1781:cluster{dbl[], dbl[]})  [unwired: 1 in]
            n1859 = Bundle "Bundle"(w1775, w1807) -> (w1918:cluster{dbl[], dbl[]})  [unwired: 1 in]
            n1860 = Bundle "Bundle"(w1775, w1803) -> (w1841:cluster{dbl[], dbl[]})  [unwired: 1 in]
            n1861 = Bundle "Bundle"(w1775, w1857) -> (w1865:cluster{dbl[], dbl[]})  [unwired: 1 in]
            n1862 = Bundle "Bundle"(w1775, w1859) -> (w1927:cluster{dbl[], dbl[]})  [unwired: 1 in]
            n1863 = Bundle "Bundle"(w1775, w1896) -> (w1909:cluster{dbl[], dbl[]})  [unwired: 1 in]
            n1864 = Bundle "Bundle"(w1805, w1801) -> (w1813:cluster{dbl[], dbl[]})  [unwired: 1 in]
            n1865 = Bundle "Bundle"(w1771, w1770) -> (w1779:cluster{dbl[], dbl[]})  [unwired: 1 in]
            n1866 = Bundle "Bundle"(w1771, w1805) -> (w1917:cluster{dbl[], dbl[]})  [unwired: 1 in]
            n1867 = Bundle "Bundle"(w1771, w1801) -> (w1839:cluster{dbl[], dbl[]})  [unwired: 1 in]
            n1868 = Bundle "Bundle"(w1771, w1855) -> (w1863:cluster{dbl[], dbl[]})  [unwired: 1 in]
            n1869 = Bundle "Bundle"(w1771, w1860) -> (w1925:cluster{dbl[], dbl[]})  [unwired: 1 in]
            n1870 = Bundle "Bundle"(w1771, w1878) -> (w1910:cluster{dbl[], dbl[]})  [unwired: 1 in]
            n1871 = call-poly <vilib>:"Mean.vi"("X"=w1858) -> ("mean"=→"CP1":dbl)  [unwired: 1 out]
            n1872 = call-poly <vilib>:"Mean.vi"("X"=w1799) -> ("mean"=→"КОФ2 3":dbl)  [unwired: 1 out]
            n1873 = call-poly <vilib>:"Mean.vi"("X"=w1857) -> ("mean"=→"CP2":dbl)  [unwired: 1 out]
            n1874 = call-poly <vilib>:"Mean.vi"("X"=w1859) -> ("mean"=→"КОФ2":dbl)  [unwired: 1 out]
            n1875 = call-poly <vilib>:"Mean.vi"("X"=w1797) -> ("mean"=→"КОФ2 5":dbl)  [unwired: 1 out]
            n1876 = call-poly <vilib>:"Mean.vi"("X"=w1855) -> ("mean"=→"CP4":dbl)  [unwired: 1 out]
            n1877 = call-poly <vilib>:"Mean.vi"("X"=w1860) -> ("mean"=→"КОФ4":dbl)  [unwired: 1 out]
            n1878 = Bundle "Bundle"(w1777, w1804) -> (w1768:cluster{dbl[], dbl[]})  [unwired: 1 in]
            n1879 = Bundle "Bundle"(w1777, w1858) -> (w1791:cluster{dbl[], dbl[]})  [unwired: 1 in]
            n1880 = Build Array "Build Array"(w1768, w1791) -> (w1794:cluster{dbl[], dbl[]}[])
            "XY Graph 17" <- w1794
            n1881 = Build Array "Build Array"(w1782, w1781, w1780, w1779) -> (→"Frequency ( Hz )":cluster{dbl[], dbl[]}[])
            n1882 = Build Array "Build Array"(w1810, w1811, w1812, w1813) -> (→"Air Temp ( °C ) vs Humidity ( % RH )":cluster{dbl[], dbl[]}[])
            n1883 = Build Array "Build Array"(w1795, w1918, w1916, w1917) -> (→"Air Temperature  ( °C )":cluster{dbl[], dbl[]}[])
            n1884 = Build Array "Build Array"(w1768, w1841, w1840, w1839) -> (→"Humidity ( %RH )":cluster{dbl[], dbl[]}[])
            n1885 = Build Array "Build Array"(w1796, w1927, w1926, w1925) -> (→"Coefficient Of Friction":cluster{dbl[], dbl[]}[])
            n1886 = Build Array "Build Array"(w1791, w1865, w1864, w1863) -> (→"Sample Temperature ( °C )":cluster{dbl[], dbl[]}[])
            n1887 = Build Array "Build Array"(w1769, w1909, w1911, w1910) -> (→"XY Graph 13":cluster{dbl[], dbl[]}[])
            n1888 = Bundle "Bundle"(w1777, w1800) -> (w1822:cluster{dbl[], dbl[]})  [unwired: 1 in]
            n1889 = Bundle "Bundle"(w1773, w1798) -> (w1820:cluster{dbl[], dbl[]})  [unwired: 1 in]
            n1890 = Bundle "Bundle"(w1775, w1799) -> (w1821:cluster{dbl[], dbl[]})  [unwired: 1 in]
            n1891 = Bundle "Bundle"(w1771, w1797) -> (w1819:cluster{dbl[], dbl[]})  [unwired: 1 in]
            n1892 = Build Array "Build Array"(w1822, w1821, w1820, w1819) -> (→"Stroke ( mm )":cluster{dbl[], dbl[]}[])
            n1893 = local write "XY Graph 16"(w1794) -> ()
          }
          frame #2 {
          }
          frame #3 {
            n1894 = local write "Numeric 8"(0 ("Numeric 8")) -> ()
            n1895 = local write "Numeric 11"(0 ("Numeric 11")) -> ()
            n1896 = local write "Numeric 12"(0 ("Numeric 12")) -> ()
            n1897 = local write "Numeric 13"(0 ("Numeric 13")) -> ()
            n1898 = property on="OPEN" class="Bool (strict)"("Visible"=TRUE) -> ()  [unwired: 2 in, 2 out]
            n1899 = local read "String Control 2"() -> (w2094:string)
            n1900 = local read "String Control 4"() -> (w2093:string)
            n1901 = local read "String Control 6"() -> (w2092:string)
            n1902 = local read "String Control 8"() -> (w2091:string)
            n1903 = Match Pattern(string=w2094, regular expression="Samples / cycle :- ") -> (after substring=w2108:string)  [unwired: 1 in, 3 out]
            n1904 = Match Pattern(string=w2094, regular expression="Frequency :- ") -> (after substring=w2127:string)  [unwired: 1 in, 3 out]
            n1905 = Match Pattern(string=w2093, regular expression="Samples / cycle :- ") -> (after substring=w2104:string)  [unwired: 1 in, 3 out]
            n1906 = Match Pattern(string=w2093, regular expression="Frequency :- ") -> (after substring=w2122:string)  [unwired: 1 in, 3 out]
            n1907 = Match Pattern(string=w2092, regular expression="Samples / cycle :- ") -> (after substring=w2100:string)  [unwired: 1 in, 3 out]
            n1908 = Match Pattern(string=w2092, regular expression="Frequency :- ") -> (after substring=w2117:string)  [unwired: 1 in, 3 out]
            n1909 = Match Pattern(string=w2091, regular expression="Samples / cycle :- ") -> (after substring=w2096:string)  [unwired: 1 in, 3 out]
            n1910 = Match Pattern(string=w2091, regular expression="Frequency :- ") -> (after substring=w2112:string)  [unwired: 1 in, 3 out]
            n1911 = String Subset(string=w2108, length (rest)=6 ("length (rest)")) -> (substring=w2110:string)  [unwired: 1 in]
            n1912 = String Subset(string=w2127, length (rest)=9 ("length (rest)")) -> (substring=w2129:string)  [unwired: 1 in]
            n1913 = String Subset(string=w2104, length (rest)=6 ("length (rest)")) -> (substring=w2106:string)  [unwired: 1 in]
            n1914 = String Subset(string=w2122, length (rest)=9 ("length (rest)")) -> (substring=w2124:string)  [unwired: 1 in]
            n1915 = String Subset(string=w2100, length (rest)=6 ("length (rest)")) -> (substring=w2102:string)  [unwired: 1 in]
            n1916 = String Subset(string=w2117, length (rest)=9 ("length (rest)")) -> (substring=w2119:string)  [unwired: 1 in]
            n1917 = String Subset(string=w2096, length (rest)=6 ("length (rest)")) -> (substring=w2098:string)  [unwired: 1 in]
            n1918 = String Subset(string=w2112, length (rest)=9 ("length (rest)")) -> (substring=w2114:string)  [unwired: 1 in]
            n1919 = Fract/Exp String To Number(string=w2110) -> (number=w2090:dbl)  [unwired: 3 in, 1 out]
            n1920 = Fract/Exp String To Number(string=w2129) -> (number=w2130:dbl)  [unwired: 3 in, 1 out]
            n1921 = Fract/Exp String To Number(string=w2106) -> (number=w2089:dbl)  [unwired: 3 in, 1 out]
            n1922 = Fract/Exp String To Number(string=w2124) -> (number=w2125:dbl)  [unwired: 3 in, 1 out]
            n1923 = Fract/Exp String To Number(string=w2102) -> (number=w2088:dbl)  [unwired: 3 in, 1 out]
            n1924 = Fract/Exp String To Number(string=w2119) -> (number=w2120:dbl)  [unwired: 3 in, 1 out]
            n1925 = Fract/Exp String To Number(string=w2098) -> (number=w2087:dbl)  [unwired: 3 in, 1 out]
            n1926 = Fract/Exp String To Number(string=w2114) -> (number=w2115:dbl)  [unwired: 3 in, 1 out]
            n1927 = local write "sample1"(w2090) -> ()
            n1928 = local write "freq1"(w2130) -> ()
            n1929 = local write "sample2"(w2089) -> ()
            n1930 = local write "freq2"(w2125) -> ()
            n1931 = local write "sample3"(w2088) -> ()
            n1932 = local write "freq3"(w2120) -> ()
            n1933 = local write "sample4"(w2087) -> ()
            n1934 = local write "freq 4"(w2115) -> ()
          }
        }
      }
    }
    n1935 = case shown="True" w1577 {
      selector: w1577 -> [_ w1706]
      frame False {
      }
      frame True {
        n1936 = Not(x=w1706) -> (.not. x?=w1702:bool)
        n1937 = local write "service 3"(w1702) -> ()
        n1938 = local write "OPEN 6"(w1702) -> ()
        n1939 = call <vilib>:"System Exec.vi"("wait until completion? (T)"=TRUE, "command line"="C:\\LAB-IQ\\Scar View.exe") -> ("error out"=→"error out 5":errorcluster)  [unwired: 6 in, 3 out]
      }
    }
    n1940 = case shown="\"Acquire\", Default" w1589 {
      frame "Acquire", Default {
        w2604 = 0.2 ("y")
        w2609 = 1.0 ("y")
        w2610 = 0.8 ("y")
        # "Elapsed time\ncof\nstroke\nAir temp\nTemp\nHumidity"
        n1941 = disable-structure shown="Disabled" {
          frame Disabled {
            n1942 = local read "Flag"() -> (w2627:dbl)
            n1943 = local read "RUN"() -> (w2624:bool)
            n1944 = Not(x=w2624) -> (.not. x?=w2623:bool)
            n1945 = Equal?(x=w2627, y=10.0) -> (x = y?=w2625:bool)
            n1946 = And(x=w2625, y=w2623) -> (x .and. y?=w2622:bool)
            n1947 = case shown="True" w2622 {
              frame False {
              }
              frame True {
                w2628 = FALSE ("Heater Button")
                n1948 = local write "Humidity"(w2628) -> ()
                n1949 = local write "Heater Button"(w2628) -> ()
              }
            }
          }
          frame Enabled {
          }
        }
        n1950 = disable-structure shown="Disabled" {
          frame Disabled {
            n1951 = case shown="True" {
              selector: _ -> [_ _]
              frame False {
              }
              frame True {
                w2719 = TRUE ("Heater")
                n1952 = local write "Humidity"(w2719) -> ()
                n1953 = local write "Heater Button"(w2719) -> ()
                n1954 = local read "TEST STANDARD"() -> (w2722:T3)
                n1955 = local read "TEST STANDARD"() -> (w2717:T3)
                n1956 = Equal?(x=w2722, y=enum16{"ASTM D6079", "ISO 12156", "Custom"}."ISO 12156" ("Test Standard")) -> (x = y?=w2720:bool)
                n1957 = Equal?(x=w2717, y=enum16{"ASTM D6079", "ISO 12156", "Custom"}."ASTM D6079" ("Test Standard")) -> (x = y?=w2716:bool)
                n1958 = case shown="True" w2720 {
                  frame False {
                  }
                  frame True {
                    n1959 = local write "Heater"(TRUE ("Heater")) -> ()
                    n1960 = local write "airtempflg"(FALSE ("airtempflg")) -> ()
                  }
                }
                n1961 = case shown="True" w2716 {
                  frame False {
                  }
                  frame True {
                    n1962 = local write "Heater"(FALSE ("Heater")) -> ()
                    n1963 = local write "airtempflg"(TRUE ("airtempflg")) -> ()
                  }
                }
              }
            }
          }
          frame Enabled {
          }
        }
        n1964 = stacked-sequence {
          frame #0 {
            n1965 = case shown="True" "RST FF" {
              frame False {
              }
              frame True {
                w2785 = 0.0 ("X Scale.Range:Maximum")
                n1966 = property on="Frictional Force ( N )" class="WFChart (strict)"("XScale.Maximum"=600.0 ("X Scale.Range:Maximum"), "XScale.Minimum"=w2785, "YScale.Maximum"=10.0 ("Y Scale.Range:Maximum"), "YScale.Minimum"=w2785) -> ()  [unwired: 2 in, 2 out]
              }
            }
          }
          frame #1 {
            n1967 = case shown="True" "RST TEMP" {
              frame False {
              }
              frame True {
                n1968 = property on="Temperature ( Deg C )" class="WFChart (strict)"("XScale.Minimum"=0.0 ("X Scale.Range:Minimum"), "XScale.Maximum"=600.0 ("X Scale.Range:Maximum"), "YScale.Minimum"=0.0 ("Y Scale.Range:Minimum"), "YScale.Maximum"=100.0 ("Y Scale.Range:Maximum")) -> ()  [unwired: 2 in, 2 out]
              }
            }
          }
          frame #2 {
            n1969 = case shown="True" "RSTCOF" {
              frame False {
              }
              frame True {
                n1970 = property on="Coefficient of Friction" class="WFChart (strict)"("XScale.Minimum"=0.0 ("X Scale.Range:Minimum"), "XScale.Maximum"=600.0 ("X Scale.Range:Maximum"), "YScale.Maximum"=1.0 ("X Scale.Range:Minimum"), "YScale.Minimum"=0.0 ("X Scale.Range:Minimum")) -> ()  [unwired: 2 in, 2 out]
              }
            }
          }
          frame #3 {
            n1971 = case shown="True" "RSTCOF 2" {
              frame False {
              }
              frame True {
                (unwired) 100.0 ("Y Scale.Range:Maximum")
                (unwired) 0.0 ("Y Scale.Range:Minimum")
                (unwired) 600.0 ("X Scale.Range:Maximum")
                (unwired) 0.0 ("X Scale.Range:Minimum")
              }
            }
          }
          frame #4 {
            n1972 = case shown="True" "RSTCOF 3" {
              frame False {
              }
              frame True {
                n1973 = property on="Electrical Contact Resistance ( % )" class="WFChart (strict)"("XScale.Minimum"=0.0 ("X Scale.Range:Minimum"), "XScale.Maximum"=600.0 ("X Scale.Range:Maximum"), "YScale.Minimum"=0.0 ("Y Scale.Range:Minimum"), "YScale.Maximum"=100.0 ("Y Scale.Range:Maximum")) -> ()  [unwired: 2 in, 2 out]
              }
            }
          }
        }
        n1974 = disable-structure shown="Disabled" {
          frame Disabled {
            n1975 = case shown="True" {
              selector: _ -> [_ _]
              frame False {
              }
              frame True {
                n1976 = local read "zflag 2"() -> (w2686:dbl)
                n1977 = local read "yflag"() -> (w2688:dbl)
                n1978 = Equal?(x=w2688, y=2.0 ("tflag")) -> (x = y?=w2690:bool)
                n1979 = Equal?(x=w2686, y=3.0 ("tflag")) -> (x = y?=w2689:bool)
                n1980 = And(x=w2690, y=w2689) -> (x .and. y?=w2684:bool)
                n1981 = case shown="True" w2684 {
                  frame False {
                  }
                  frame True {
                    w2715 = 0.0 ("zflag")
                    n1982 = local write "zflag"(w2715) -> ()
                    n1983 = local write "zflag 2"(w2715) -> ()
                    n1984 = Delete(path (use dialog)=path "C:/LAB-IQ-NXT/WO 2449 TT.sig" ("file path (dialog if empty)")) -> (deleted path=w2714:path)  [unwired: 4 in, 2 out]
                    n1985 = Delete(path (use dialog)=path "C:/LAB-IQ-NXT/WO 2449 TRH.sig" ("file path (dialog if empty)")) -> (deleted path=w2709:path)  [unwired: 4 in, 2 out]
                    n1986 = local read "SEN.RUN HRS"() -> (w2701:dbl)
                    n1987 = local read "SENSOR TIME"() -> (w2699:dbl)
                    n1988 = call <vilib>:"compatOverwrite.vi"("overwrite (F)"=TRUE) -> ("overwrite?"=w2691:T25)
                    n1989 = call <vilib>:"compatOverwrite.vi"("overwrite (F)"=TRUE) -> ("overwrite?"=w2695:T25)
                    n1990 = local read "Total No. of Tests"() -> (w2702:dbl)
                    n1991 = Add(x=w2699, y=w2701) -> (x+y=w2700:dbl)
                    "SEN.RUN HRS" <- w2700
                    n1992 = Open/Create/Replace File(file path (use dialog)=w2714, operation (0:open)=w2691) -> (refnum out=w2692:refnum<file>, error out=w2693:errorcluster)  [unwired: 4 in, 1 out]
                    n1993 = Open/Create/Replace File(file path (use dialog)=w2709, operation (0:open)=w2695) -> (refnum out=w2696:refnum<file>, error out=w2697:errorcluster)  [unwired: 4 in, 1 out]
                    n1994 = Deny Access(4:w2693, 6:T23."deny none" ("deny mode (2)"), 7:w2692) -> (3:w2713:refnum<file>)  [unwired: 1 out]
                    n1995 = Deny Access(4:w2697, 6:T23."deny none" ("deny mode (2)"), 7:w2696) -> (3:w2705:refnum<file>)  [unwired: 1 out]
                    n1996 = Number To Decimal String(number=w2702) -> (decimal integer string=w2710:string)  [unwired: 1 in]
                    n1997 = Number To Decimal String(number=w2700) -> (decimal integer string=w2706:string)  [unwired: 1 in]
                    n1998 = Write to Binary File(file (use dialog)=w2713, data=w2710, 5:FALSE ("prepend array or string size? (T)")) -> ()  [unwired: 3 in, 3 out]
                    n1999 = Write to Binary File(file (use dialog)=w2705, data=w2706, 5:FALSE ("prepend array or string size? (T)")) -> ()  [unwired: 3 in, 3 out]
                  }
                }
              }
            }
          }
          frame Enabled {
          }
        }
        n2000 = local read "RUN"() -> (w2613:bool)
        n2001 = local read "run replace"() -> (w2617:bool)
        n2002 = local read "run replace"() -> (w2616:bool)
        n2003 = case shown="True" w2613 {
          frame False {
            n2004 = local write "run replace"(FALSE ("run replace")) -> ()
          }
          frame True {
            "run replace" <- TRUE ("run replace")
          }
        }
        n2005 = local read "RUN"() -> (w2621:bool)
        n2006 = local read "Set Temp"() -> (w2583:dbl)
        n2007 = local read "SetTemp"() -> (w2585:dbl)
        n2008 = case shown="False" w2621 {
          tunnel: [FALSE ("TEST RUNNING") TRUE ("TEST RUNNING")] -> w2620
          frame False {
            w2804 = 0.0 ("Flag")
            n2009 = local write "Elapsed time"(0.0 ("elapsedtime")) -> ()
            n2010 = local write "Time Remaining"(w2804) -> ()
            n2011 = local write "Flag"(w2804) -> ()
            n2012 = local write "Remaining Time"(w2804) -> ()
          }
          frame True {
            n2013 = local write "Flag"(10.0 ("Flag")) -> ()
          }
        }
        n2014 = case shown="False" w2617 {
          frame False {
            n2015 = local read "zflag"() -> (→"zflag 2":dbl)
            n2016 = local write "yflag"(2.0 ("tflag")) -> ()
            n2017 = local write "FLAG 4"(0.0 ("FLAG")) -> ()
          }
          frame True {
            n2018 = local write "yflag"(1.0 ("tflag")) -> ()
            n2019 = local write "zflag"(3.0 ("zflag")) -> ()
          }
        }
        n2020 = local read "acq 2"() -> (w2615:bool)
        n2021 = local read "AIR TEMP"() -> (w2578:dbl)
        n2022 = local read "Amb temp"() -> (w2582:dbl)
        n2023 = case shown="True" "Save & Continue" {
          frame False {
          }
          frame True {
            "acq 2" <- TRUE ("acq 2")
          }
        }
        n2024 = local read "Set Rh"() -> (w2584:dbl)
        n2025 = Add(x=w2585, y=w2610) -> (x+y=w2611:dbl)
        n2026 = Subtract(x=w2585, y=w2610) -> (x-y=w2612:dbl)
        n2027 = Add(x=w2583, y=w2604) -> (x+y=w2605:dbl)
        n2028 = Subtract(x=w2583, y=w2604) -> (x-y=w2606:dbl)
        n2029 = And(x=w2615, y=w2616) -> (x .and. y?=w2614:bool)
        n2030 = Greater Or Equal?(x=w2578, y=15.0) -> (x >= y?=w2579:bool)
        "powstat" <- w2579
        n2031 = local read "Humidity ( %RH )"() -> (w2581:dbl)
        n2032 = case shown="True" "Save & Continue" {
          frame False {
          }
          frame True {
            n2033 = while {
              tunnel: "0123456789abcdefghijklmnopqrstuvwxyzABCDEFGHIJKLMNOPQRSTUVWXYZ" ("string 2") -> [w2775]
              shift-right: [w2773] -> w2768
              shift-left: "" -> [w2772]
              i -> [w2782]
              stop <- w2781 stop-if-true
              n2034 = Random Number (0-1)() -> (number: 0 to 1=w2776:dbl)
              n2035 = Multiply(x=w2776, y=62.0) -> (x*y=w2778:dbl)
              n2036 = Decrement(x="Length") -> (x-1=w2771:i16)
              n2037 = To Word Integer(number=w2778) -> (16bit integer=w2779:i16)
              n2038 = String Subset(string=w2775, offset (0)=w2779, length (rest)=1 ("length (rest)")) -> (substring=w2774:string)
              n2039 = Greater Or Equal?(x=w2782, y=w2771) -> (x >= y?=w2781:bool)
              n2040 = Concatenate Strings(w2774, w2772) -> (w2773:string)
            }
            n2041 = local write "UUID"(w2768) -> ()
          }
        }
        n2042 = In Range and Coerce(upper limit=w2611, x=w2582, lower limit=w2612) -> (In Range?=w2601:bool)  [unwired: 1 out]
        n2043 = Add(x=w2584, y=w2609) -> (x+y=w2608:dbl)
        n2044 = Subtract(x=w2584, y=w2609) -> (x-y=w2607:dbl)
        n2045 = local read "TEMP"() -> (w2580:dbl)
        n2046 = case shown="True" "Save & Continue" {
          frame False {
          }
          frame True {
            n2047 = local read "Operator ID"() -> (w3080:string)
            n2048 = local read "FILE"() -> (w3086:string)
            n2049 = String Length(string=w3086) -> (length=w3084:i32)
            n2050 = String Length(string=w3080) -> (length=w3081:i32)
            n2051 = Greater?(x=w3084, y=0) -> (0:w3083:bool)
            n2052 = Greater?(x=w3081, y=0) -> (0:w3079:bool)
            n2053 = And(x=w3083, y=w3079) -> (x .and. y?=w3078:bool)
            n2054 = case shown="True" w3078 {
              frame False {
                n2055 = stacked-sequence {
                  frame #0 {
                    n2056 = One Button Dialog(message="Please Enter a File Name and Operator ID to save data !", button name ("OK")="Ok") -> ()  [unwired: 1 out]
                  }
                  frame #1 {
                    n2057 = local write "Save & Continue"(FALSE ("OK Button")) -> ()
                  }
                }
                n2058 = local write "Save & Continue"(FALSE ("OK Button")) -> ()
              }
              frame True {
                n2059 = stacked-sequence {
                  frame #0 {
                    n2060 = local read "FILE"() -> (w3092:string)
                    n2061 = call "file check.vi"("file name in"=w3092) -> ("file name out"=w3091:string)  [unwired: 9 in, 1 out]
                    n2062 = call <vilib>:"Application Directory.vi"() -> ("Application Directory"=w3102:path)
                    n2063 = Build Path(base path=w3102, name or relative path="data") -> (appended path=w3101:path)
                    n2064 = call <vilib>:"Trim Whitespace.vi"("string"=w3091) -> ("trimmed string"=w3099:string)  [unwired: 1 in]
                    n2065 = call <vilib>:"Trim Whitespace.vi"("string"=w3091) -> ("trimmed string"=w3100:string)  [unwired: 1 in]
                    n2066 = List Folder(path=w3101) -> (folder names=w3097:string[])  [unwired: 3 in, 3 out]
                    n2067 = Match Pattern(string=w3099, regular expression="_(") -> (before substring=w3096:string)  [unwired: 1 in, 3 out]
                    n2068 = for {
                      tunnel: w3097 -> [w3111] mode=indexing
                      tunnel: w3096 -> [w3109]
                      shift-right: [w3107] -> w3094
                      shift-left: bool[] [] -> [w3108]
                      n2069 = Match Pattern(string=w3111, regular expression="_(") -> (before substring=w3110:string)  [unwired: 1 in, 3 out]
                      n2070 = Equal?(x=w3110, y=w3109) -> (x = y?=w3106:bool)
                      n2071 = case shown="True" w3106 {
                        tunnel: w3106 -> [_ w3114]
                        tunnel: w3108 -> [w3113 w3116]
                        tunnel: [w3113 w3115] -> w3107
                        frame False {
                        }
                        frame True {
                          n2072 = Insert Into Array(array=w3116, new element=w3114) -> (w3115:bool[])  [unwired: 1 in]
                        }
                      }
                    }
                    n2073 = Equal?(x=w3097, y=w3096) -> (x = y?=w3105:bool[])
                    n2074 = Or Array Elements(Boolean array=w3105) -> (logical OR=w3104:bool)
                    n2075 = Array Size(array=w3094) -> (size(s)=w3093:i32)
                    n2076 = case shown="True" w3104 {
                      tunnel: w3100 -> [_ w3124]
                      tunnel: w3093 -> [_ w3117]
                      frame False {
                      }
                      frame True {
                        n2077 = Number To Decimal String(number=w3117) -> (decimal integer string=w3120:string)  [unwired: 1 in]
                        n2078 = Search/Split String(string=w3124, search string/char (-)="_(" ("regular expression")) -> (substring before match=w3122:string)  [unwired: 1 in, 2 out]
                        n2079 = Concatenate Strings(w3122, "_(" ("regular expression"), w3120, ")" ("regular expression")) -> (w3118:string)
                        n2080 = local write "FILE"(w3118) -> ()
                      }
                    }
                  }
                  frame #1 {
                    w3126 = 0.0
                    w3139 = cluster{"y":dbl, dbl, "y":dbl}[] [] ("History Data")
                    w3140 = FALSE ("Heater Button")
                    (unwired) ")!" ("string")
                    (unwired) ")" ("string")
                    w3138 = dbl[] [] ("History Data")
                    w3144 = "\r"
                    # "C:\\WinDucom\\Data\\"
                    # "C:\\LAB-IQ-NXT\\data"
                    n2081 = local write "Humidity ( %RH )"(w3126) -> ()
                    n2082 = local write "Frequency ( Hz )"(w3126) -> ()
                    n2083 = local write "Stroke 3"(w3126) -> ()
                    n2084 = local write "speedop"(0.0 ("PIDclk 2")) -> ()
                    n2085 = local write "Set Temp 2"(65.0 ("Set Temp 2")) -> ()
                    n2086 = local write "AIR TEMP"(w3126) -> ()
                    n2087 = local write "clk"(0.0 ("clk")) -> ()
                    n2088 = local write "Stroke 4"(w3126) -> ()
                    n2089 = local write "COF 2"(w3126) -> ()
                    n2090 = local write "TEMP"(w3126) -> ()
                    n2091 = local write "ecr 3"(w3126) -> ()
                    n2092 = local write "FF 3"(w3126) -> ()
                    n2093 = local write "FF 2"(w3126) -> ()
                    n2094 = property on="Humidity ( %RH )" class="WFChart (strict)"("History Data"=w3138) -> ()  [unwired: 2 in, 2 out]
                    n2095 = property on="Coefficient of Friction" class="WFChart (strict)"("History Data"=w3138) -> ()  [unwired: 2 in, 2 out]
                    n2096 = property on="Coefficient of Friction" class="WFChart (strict)"("History Data"=w3138) -> ()  [unwired: 2 in, 2 out]
                    n2097 = property on="Frictional Force ( N )" class="WFChart (strict)"("History Data"=w3138) -> ()  [unwired: 2 in, 2 out]
                    n2098 = property on="Electrical Contact Resistance ( % )" class="WFChart (strict)"("History Data"=w3138) -> ()  [unwired: 2 in, 2 out]
                    n2099 = property on="Electrical Contact Resistance ( % )" class="WFChart (strict)"("History Data"=w3138) -> ()  [unwired: 2 in, 2 out]
                    n2100 = property on="Temperature ( Deg C )" class="WFChart (strict)"("History Data"=w3138) -> ()  [unwired: 2 in, 2 out]
                    n2101 = property on="Frictional Force ( N )" class="WFChart (strict)"("History Data"=w3138) -> ()  [unwired: 2 in, 2 out]
                    n2102 = property on="Coefficient of Friction" class="WFChart (strict)"("History Data"=w3138) -> ()  [unwired: 2 in, 2 out]
                    n2103 = property on="Frictional Force ( N )" class="WFChart (strict)"("History Data"=w3138) -> ()  [unwired: 2 in, 2 out]
